vi "CleanUp.vi"(0 "ActionBeep in":refnum<class "ActionBeep.lvclass">, 5 "error in (no error)":errorcluster) -> (14 "ActionBeep out":refnum<class "ActionBeep.lvclass">, 19 "error out":errorcluster)   [LabVIEW 2017, in "ActionBeep.lvclass"]
doc: "Base class implementation (empty)."
uses:
  ActionBeep.lvclass
  <vilib>/Waveform/WDTOps.llb/WDT Append Waveforms DBL.vi
  <vilib>/measure/NI_MABase.lvlib
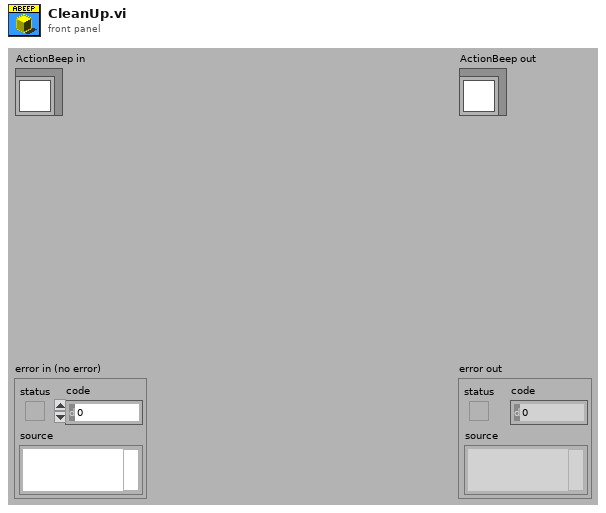
[diagram p1: front panel]
types:
  T1 = enum16{"Sine Wave", "Triangle Wave", "Square Wave", "Sawtooth Wave"}
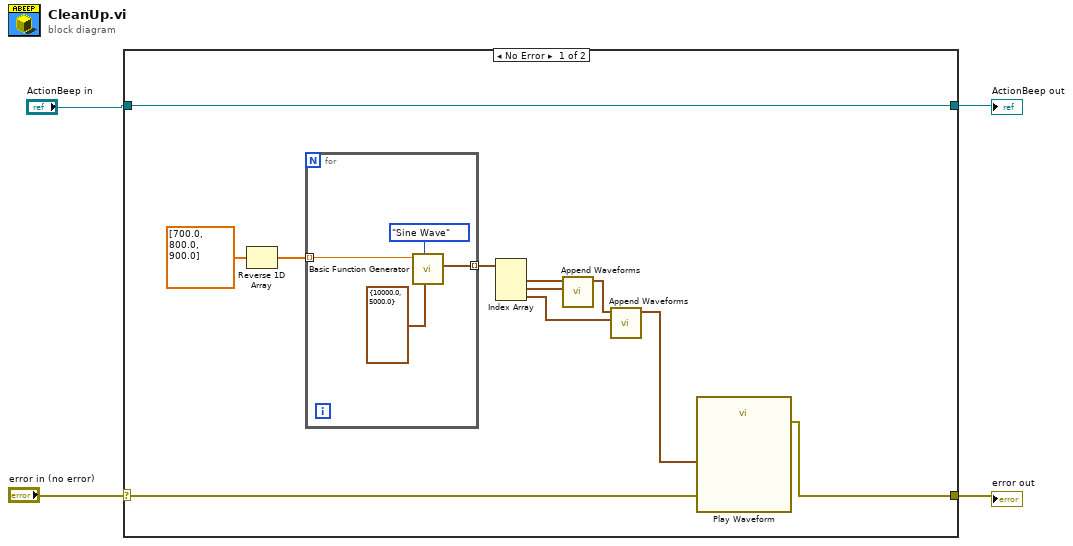
[diagram p0: block diagram]
diagram:
  n1 = case shown="No Error" "error in (no error)" {
    selector: "error in (no error)" -> [w6 w20]
    tunnel: "ActionBeep in" -> [w15 w21]
    tunnel: [w15 w21] -> w2
    tunnel: [w5 w20] -> w1
    frame No Error {
      n2 = Reverse 1D Array(array=dbl[] [700.0, 800.0, 900.0]) -> (reversed array=w7:dbl[])
      n3 = for {
        tunnel: [w17] -> w13 mode=indexing
        tunnel: w7 -> [w16] mode=indexing
        n4 = call <vilib>:"Basic Function Generator.vi"("sampling info"=cluster{"Fs":dbl, "#s":dbl} {"Fs"=10000.0, "#s"=5000.0}, "signal type"=T1."Sine Wave", "frequency"=w16) -> ("signal out"=w17:waveform(dbl))  [unwired: 6 in, 2 out]
      }
      n5 = Index Array(array=w13) -> (element #1=w12:waveform(dbl), element #2=w11:waveform(dbl), element #3=w9:waveform(dbl))  [unwired: 3 in]
      n6 = call-poly <vilib>:"Append Waveforms.vi"("waveform B"=w11, "waveform A"=w12) -> ("waveform out"=w10:waveform(dbl))  [unwired: 8 in, 1 out]
      n7 = call-poly <vilib>:"Append Waveforms.vi"("waveform B"=w9, "waveform A"=w10) -> ("waveform out"=w8:waveform(dbl))  [unwired: 8 in, 1 out]
      n8 = call "Play Waveform"("Data"=w8, "error in"=w6) -> ("error out"=w5:errorcluster)  [unwired: 17 in]
    }
    frame Error {
    }
  }
  "error out" <- w1
  "ActionBeep out" <- w2
